vi "StockFPGA_PlugInOptionalWaitOnIrq.vi"(0 "session in":T1, 5 "interrupt number(s) mask":u32 format="%.0x", 7 "timeout in ms":i32, 11 "error in (no error)":errorcluster) -> (4 "session out":T1, 6 "interrupt received?":bool, 8 "status register if irq received":u32, 10 "timed out?":bool, 15 "error out":errorcluster)   [LabVIEW 2017]
uses:
  niFpgaHostInterfaceSession.ctl
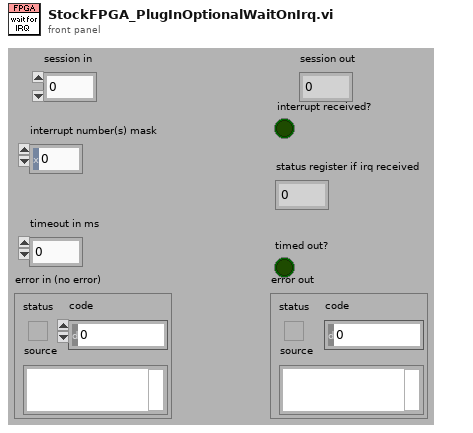
[diagram p1: front panel]
types:
  T1 = typedef "niFpgaHostInterfaceSession.ctl" = u32
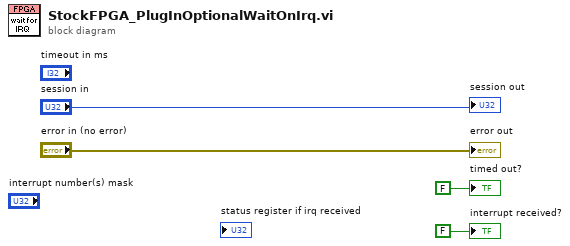
[diagram p0: block diagram]
diagram:
  "error out" <- "error in (no error)"
  "session out" <- "session in"
  "interrupt received?" <- FALSE ("interrupt received?")
  "timed out?" <- FALSE ("timed out?")
